vi "Set Spur Evaluations.vi"(8 "error in (no error)":errorcluster, 10 "Step In":refnum<k7>, 11 "Skyworks Spur Test in":refnum<class "Skyworks Spur Test.lvclass">) -> (0 "error out":errorcluster, 2 "Step Out":refnum<k7>, 3 "Skyworks Spur Test out":refnum<class "Skyworks Spur Test.lvclass">)   [LabVIEW 2018, in "Skyworks Spur Test.lvlib" / "Skyworks Spur Test.lvclass"]
uses:
  Skyworks Spur Test.lvclass
  C:/Sequence Automation/Plugins/Measurement Interface.lvlibp/Measurement Interface.lvclass
  Skyworks Spur Test.lvclass/Skyworks Spur Test.ctl
  Read SG Parameters.vi
  Plugins/Measurement Interface.lvlibp/Private Methods/Engine Reference/Read Engine Reference.vi
  Plugins/Measurement Interface.lvlibp/Private Methods/Measurement Name/Read Measurement Name.vi
  Plugins/Measurement Interface.lvlibp/Private Methods/Measurement Parameters/Read Measurement Parameters.vi
  <vilib>/Analysis/1siggen.llb/Ramp Pattern by Delta.vi
  Plugins/String Database.lvlibp/String Database.lvclass
  Evaluations/Skyworks/SpurTest/Skyworks_SpurTest.lvclass
  <vilib>/Analysis/NI_AALBase.lvlib
  Plugins/TestStand API Tools (TSAT).lvlibp/Step Actions/TSAT Step Actions.lvlib
  Plugins/Test Number and Bin Generator.lvlibp/Test Number and Bin Generator/Test Number and Bin Generator.lvclass
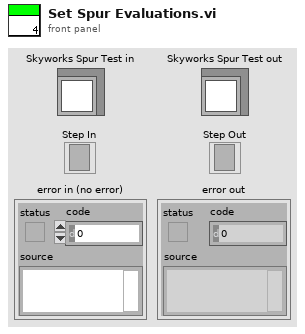
[diagram p1: front panel]
types:
  T1 = cluster{"Start Frequency":dbl, "Stop Frequency":dbl, "Delta":dbl}
  T2 = typedef "TestStand API Tools (TSAT).lvlibp/TSAT Evaluation Actions.lvlib/TSAT Evaluation.ctl" = cluster{"Test Name":string, "Pin":string, "Units":string, "SI Scaling":T3, "Test Number":i32, "Published Data Id":string, "Low Limit":dbl, "High Limit":dbl, "Export Data Location":string, "Software Bin":i64, "Evaluation Type":T4, "Test Data Source":string}
  T3 = typedef "TestStand API Tools (TSAT).lvlibp/TSAT Evaluation Actions.lvlib/TSAT Eval SI Unit Scaling.ctl" = i16
  T4 = typedef "TestStand API Tools (TSAT).lvlibp/TSAT Evaluation Actions.lvlib/TSAT Evaluation Type.ctl" = enum16{"Numeric Limit", "Pass/Fail", "None"}
  T5 = typedef "Test Number and Bin Generator.lvlibp/Test Number and Bin Generator.lvclass/Session Handle.ctl" = refnum<data-value>
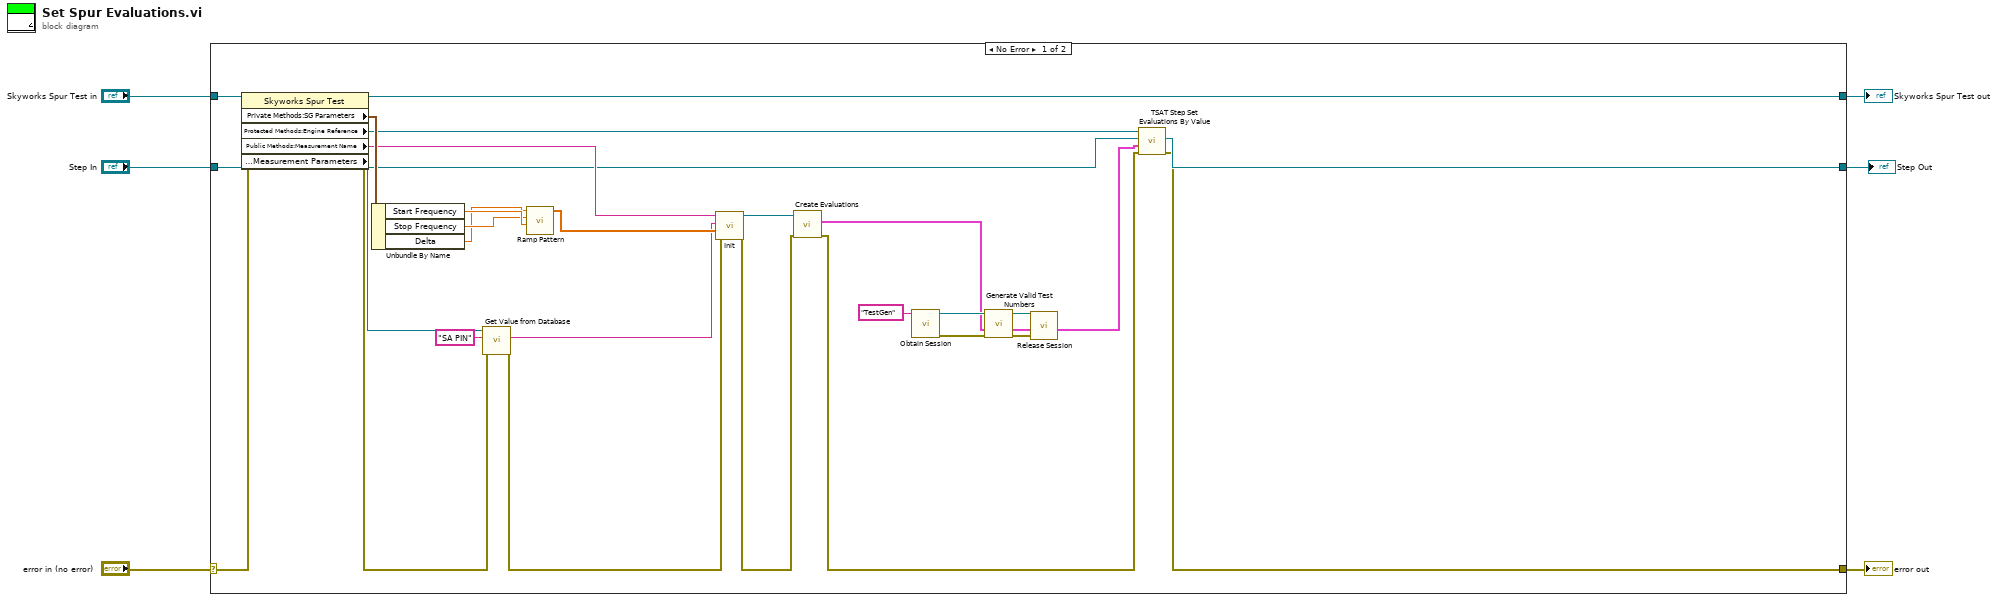
[diagram p0: block diagram]
diagram:
  n1 = case shown="No Error" "error in (no error)" {
    selector: "error in (no error)" -> [w34 w37]
    tunnel: [w14 w37] -> w5
    tunnel: [w32 w36] -> w3
    tunnel: "Skyworks Spur Test in" -> [w33 w36]
    tunnel: "Step In" -> [w17 w35]
    tunnel: [w16 w35] -> w1
    frame No Error {
      n2 = property class="Skyworks Spur Test"(reference=w33, error in=w34) -> (reference out=w32:refnum<class "Skyworks Spur Test.lvclass">, error out=w24:errorcluster, "Private Methods:SG Parameters"=w31:T1, "Protected Methods:Engine Reference"=w18:refnum<k7>, "Public Methods:Measurement Name"=w26:string, "Protected Methods:Measurement Parameters"=w25:refnum<class "String Database.lvclass">)
      n3 = Unbundle By Name(w31) -> ("Start Frequency"=w30:dbl, "Stop Frequency"=w29:dbl, "Delta"=w28:dbl)
      n4 = call "Get Value from Database.vi"("error in (no error)"=w24, "Entry Name"="SA PIN", "Message in"=w25) -> ("error out"=w23:errorcluster, "Entry Value"=w21:string)  [unwired: 5 in, 2 out]
      n5 = call-poly <vilib>:"Ramp Pattern.vi"("start"=w30, "end"=w29, "delta"=w28) -> ("Ramp Pattern"=w27:dbl[])  [unwired: 6 in, 2 out]
      n6 = call "Init.vi"("error in (no error)"=w23, "Frequencies"=w27, "SA Pin"=w21, "Measurement Name"=w26) -> ("error out"=w19:errorcluster, "Skyworks_SpurTest out"=w20:refnum<class "Skyworks_SpurTest.lvclass">)  [unwired: 6 in]
      n7 = call-dynamic "Create Evaluations.vi"("error in (no error)"=w19, "IEvaluation in"=w20) -> ("error out"=w15:errorcluster, "Evaluations Out"=w10:T2[])  [unwired: 7 in, 1 out]
      n8 = call "Obtain Session.vi"("Session  Name ()"="TestGen") -> ("Session Handle"=w12:T5, "error out"=w11:errorcluster)  [unwired: 13 in]
      n9 = call "Generate Valid Test Numbers.vi"("Session Handle in"=w12, "Evaluations In"=w10, "error in (no error)"=w11) -> ("Session Handle out"=w8:T5, "Evaluations Out"=w9:T2[], "error out"=w7:errorcluster)  [unwired: 10 in]
      n10 = call "Release Session.vi"("Session Handle"=w8, "error in (no error)"=w7) -> ()  [unwired: 13 in, 1 out]
      n11 = call "TSAT Step Set Evaluations By Value.vi"("Error In"=w15, "Evaluation Data"=w9, "Step In"=w17, "Engine In"=w18) -> ("Error Out"=w14:errorcluster, "Step Out"=w16:refnum<k7>)  [unwired: 5 in, 1 out]
    }
    frame Error {
    }
  }
  "error out" <- w5
  "Skyworks Spur Test out" <- w3
  "Step Out" <- w1
